vi "New-Engine.vi"(8 "error in (no error)":errorcluster) -> (0 "error out":errorcluster, 3 "Engine":refnum<class "Engine.lvclass">)   [LabVIEW 2024, in "GLF.lvlib" / "Engine.lvclass"]
uses:
  Engine.lvclass
  Engine.lvclass/Engine.ctl
  Core.vi
  IAmGLF/IAmGLF.lvclass
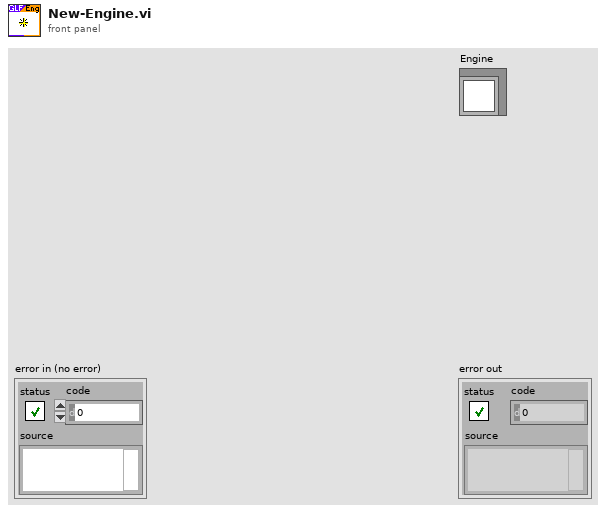
[diagram p1: front panel]
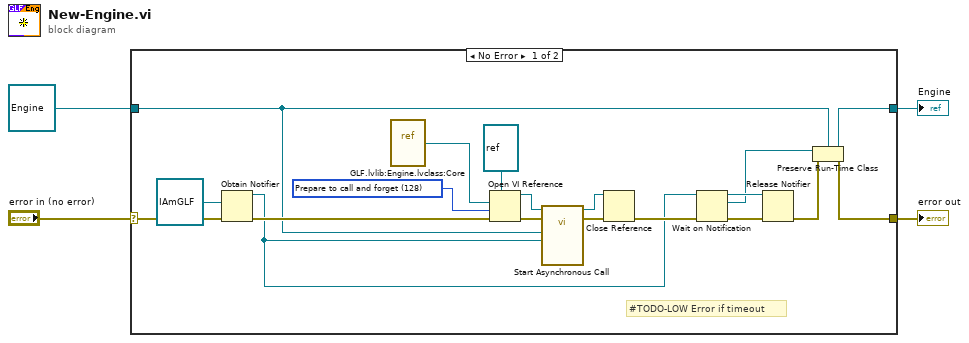
[diagram p0: block diagram]
diagram:
  n1 = case shown="No Error" "error in (no error)" {
    selector: "error in (no error)" -> [w20 w25]
    tunnel: [w19 w25] -> w3
    tunnel: [w8 w24] -> w1
    tunnel: refnum<class "Engine.lvclass"> refnum ("Engine in") -> [w7 w24]
    frame No Error {
      w12 = 128 items=["Record modifications"=1, "Open templates for editing"=2, "Prompt user to save"=4, "Prepare for reentrant run"=8, "Prompt to find missing subVIs"=16, "Hide loading dialog box"=32, "Enable simultaneous calls"=64, "Prepare to call and forget"=128, "Simultaneous call and forget"=192, "Prepare to call and collect"=256, "Simultaneous call and collect"=320]
      # "#TODO-LOW Error if timeout"
      n2 = Obtain Notifier(notification data type=refnum<class "IAmGLF.lvclass"> refnum ("notification"), error in (no error)=w20) -> (notifier out=w9:refnum<notifier>, error out=w11:errorcluster)  [unwired: 2 in, 1 out]
      n3 = vi-ref "GLF.lvlib:Engine.lvclass:Core.vi"() -> (w14:refnum<vi>)
      n4 = Open VI Reference(type specifier VI Refnum (for type only)=refnum<vi> refnum, vi path=w14, options=w12, error in (no error)=w11) -> (vi reference=w16:refnum<vi>, error out=w18:errorcluster)  [unwired: 2 in]
      n5 = call-by-ref "Start Asynchronous Call"(reference=w16, error in=w18, "Class Return Notifier"=w9, "Engine in"=w7) -> (reference out=w15:refnum<vi>, error out=w17:errorcluster)  [unwired: 10 in]
      n6 = Close Reference(reference=w15, error in (no error)=w17) -> (error out=w10:errorcluster)
      n7 = Wait on Notification(notifier=w9, error in (no error)=w10) -> (notifier out=w23:refnum<notifier>, notification=w6:refnum<class "IAmGLF.lvclass">, error out=w22:errorcluster)  [unwired: 2 in, 1 out]
      n8 = Release Notifier(notifier=w23, error in (no error)=w22) -> (error out=w21:errorcluster)  [unwired: 1 in, 2 out]
      n9 = Preserve Run-Time Class(object in=w6, error in=w21, 2:w7) -> (object out=w8:refnum<class "Engine.lvclass">, error out=w19:errorcluster)
    }
    frame Error {
    }
  }
  "error out" <- w3
  "Engine" <- w1
